vi "Write data.vi"(8 "error in (no error)":errorcluster, 9 "Operator":string, 10 "table name":string="Test_Results", 11 "connection reference":T1) -> (0 "error out":errorcluster, 3 "connection reference out":T1)   [LabVIEW 2018]
doc: "The T1 Parametric testing application performs parametric testing of T1 signals. The T1 signal is a 1.544 Mb/s pulsed digital signal formed by multiplexing 24 voice channels. Each channel is sampled at 8000 samples/sec. Each sample is then converted to 8 bits using Pulse Coded Multiplexing. The 24 channels are then time-division multiplexed. Each frame, which corresponds to one sampling period, contains 192 bits ( 8 times 24) plus one bit for frame synchronization. Since frames occur at 8000 times per second, the bit rate is 1.544 Mb/s\n\nThis application performs the following parametric tests on T1 signals:\n\n1. Mask Test: Compares T1 signals with standard masks. The type of masks that are supported are ITU G.703 mask, EIA/TIA 547 and ANSI T1.102. The graph shows the mask in grey, the actual signal in green and failures as red squares. A boolean indicates whether the signal passed or failed the mask test and the indicator Number of Hits shows the number of times the signal did not pass the mask test.\n\n2. Measure T1 signal amplitude : Measures the amplitude of the T1 signal. The peak amplitude is displayed in the indicator Measured Amplitude.\n\n3. Measure T1 signal frequency : Measures the frequency of the T1 signal. The signal frequency in MHz is displayed in the indicator Measured Frequency."
uses:
  <vilib>/addons/database/Connection.llb/Conn ObjectReference.ctl
  <vilib>/addons/database/Auxilliary.llb/DB Tools Column Info.ctl
  <vilib>/addons/database/Auxilliary.llb/DB Tools DataTypes.ctl
  <vilib>/addons/database/NI_Database_API.lvlib
panel:
  in  "Log to Database":bool
  in  "quit":bool
  # "Telecommunications Parametric Testing"
  # "Instructions: Click Start Testing, then Log to Database, then Quit."
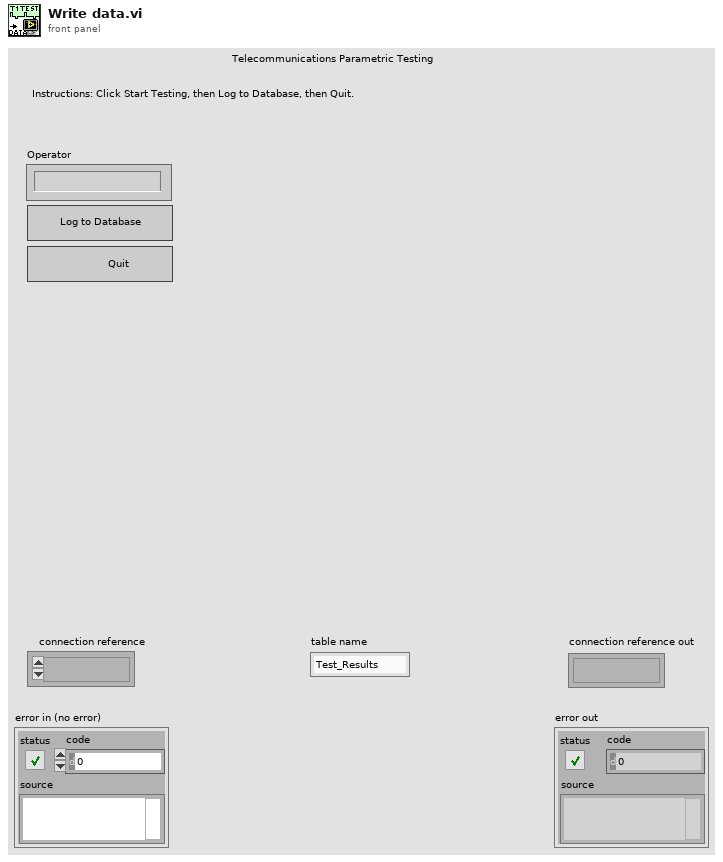
[diagram p1: front panel]
types:
  T1 = typedef "NI_Database_API.lvlib/Conn ObjectReference.ctl" = refnum<k1>
  T2 = enum8{"Enabled", "Disabled", "Disabled and Grayed Out"}
  T3 = typedef "NI_Database_API.lvlib/DB Tools Column Info.ctl" = cluster{"column name":string, "data type":T4, "size":i32, "allow null?":bool}
  T4 = typedef "NI_Database_API.lvlib/DB Tools DataTypes.ctl" = enum16{"String", "Long (I32)", "Single (SGL)", "Double (DBL)", "Date/Time", "Binary"}
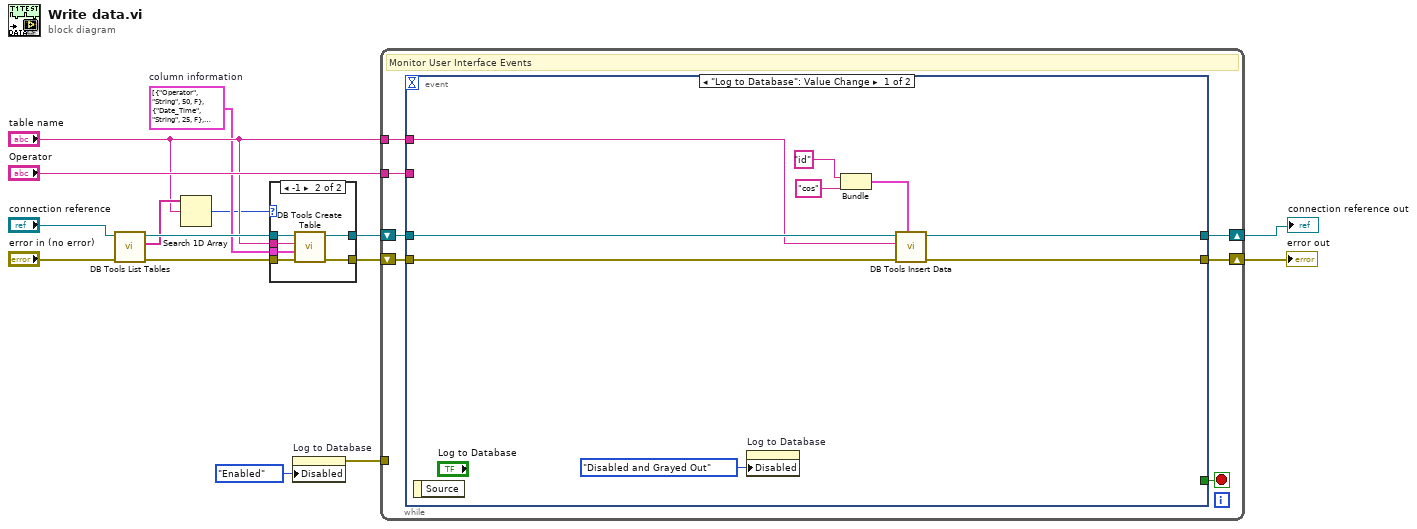
[diagram p0: block diagram]
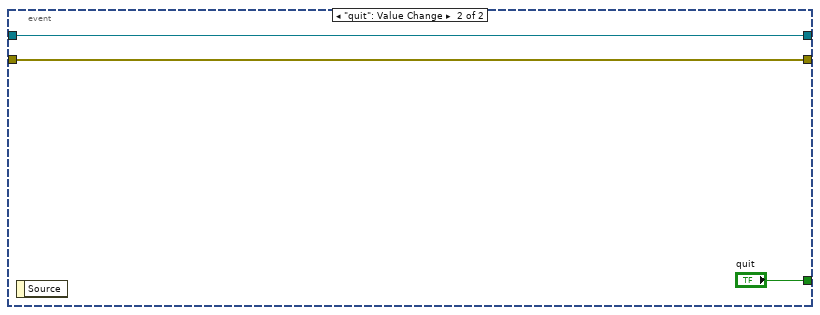
[diagram p3: hidden frame]
diagram:
  w4 = T3[] [{"column name"="Operator", "data type"=enum."String", "size"=50, "allow null?"=FALSE}, {"column name"="Date_Time", "data type"=enum."String", "size"=25, "allow null?"=FALSE}, {"column name"="UUT_Serial_Num", "data type"=enum."String", "size"=13, "allow null?"=FALSE}, {"column name"="Pass_Fail", "data type"=enum."String", "size"=4, "allow null?"=FALSE}, {"column name"="Frequency", "data type"=enum."Double (DBL)", "size"=0, "allow null?"=FALSE}, {"column name"="Polarity", "data type"=enum."String", "size"=8, "allow null?"=FALSE}, {"column name"="Standard", "data type"=enum."String", "size"=9, "allow null?"=FALSE}]  # column information
  n1 = call <vilib>:"DB Tools List Tables.vi"("error in (no error)"="error in (no error)", "connection reference"="connection reference") -> ("error out"=w11:errorcluster, "tables"=w8:string[], "connection reference out"=w9:T1)  [unwired: 3 in]
  n2 = Search 1D Array(1D array=w8, element="table name") -> (index of element=w3:i32)  [unwired: 1 in]
  n3 = case shown="-1" w3 {
    tunnel: w11 -> [w16 w23]
    tunnel: w9 -> [w17 w22]
    tunnel: "table name" -> [_ w21]
    tunnel: [w16 w20] -> w6
    tunnel: [w17 w19] -> w5
    tunnel: w4 -> [_ w18]
    frame Default {
    }
    frame -1 {
      n4 = call <vilib>:"DB Tools Create Table.vi"("error in (no error)"=w23, "column information"=w18, "table"=w21, "connection reference"=w22) -> ("error out"=w20:errorcluster, "connection reference out"=w19:T1)  [unwired: 4 in]
    }
  }
  n5 = property on="Log to Database" class="Bool"("Disabled"=T2."Enabled") -> (error out=w2:errorcluster)  [unwired: 2 in, 1 out]
  n6 = while {
    shift-right: [w27] -> w14
    shift-left: w5 -> [w26]
    shift-right: [w28] -> w15
    shift-left: w6 -> [w29]
    tunnel: "Operator" -> [w25]
    tunnel: "table name" -> [w24]
    tunnel: w2 -> [_]
    stop <- w30 stop-if-true
    # "Monitor User Interface Events"
    n7 = event shown="[0] \"Log to Database\": Value Change" {
      selector: _ -> [_ _]
      dyn-events: _ -> [_ _]
      timeout: _ -> [_ _]
      tunnel: [_ "quit"] -> w30
      tunnel: w29 -> [w39 w40]
      tunnel: [w38 w40] -> w28
      tunnel: [w37 w41] -> w27
      tunnel: w26 -> [w36 w41]
      tunnel: w25 -> [_ _]
      tunnel: w24 -> [w34 _]
      event "Log to Database": Value Change {
        n8 = event-data() -> ()  [unwired: 1 in, 1 out]
        n9 = property on="Log to Database" class="Bool"("Disabled"=T2."Disabled and Grayed Out") -> ()  [unwired: 2 in, 2 out]
        n10 = Bundle("id", "cos") -> (w33:cluster{string, string})  [unwired: 1 in]
        n11 = call <vilib>:"DB Tools Insert Data.vi"("data"=w33, "error in (no error)"=w39, "table"=w34, "connection reference"=w36) -> ("error out"=w38:errorcluster, "connection reference out"=w37:T1)  [unwired: 6 in]
      }
      event "quit": Value Change {
        n12 = event-data() -> ()  [unwired: 1 in, 1 out]
      }
    }
  }
  "connection reference out" <- w14
  "error out" <- w15
